vi "qc5psm.vi"() -> ()   [LabVIEW 2020]
uses:
  <instrlib>/CAEN PSM/CAEN PSM.lvlib
panel:
  in  "Tab Control":enum32{"Page 1"}(tab)
  in  "VISA resource name":refnum<visa-resource-name>
  in  "Serial Configuration":T1={"Baud Rate"=9600, "Parity"=enum."None", "Data Bits"=8, "Stop Bits"=10, "Flow Control"=0} {"Flow Control" items=["None", "XON/XOFF", "RTS/CTS", "XON/XOFF & RTS/CTS", "DTR/DSR", "XON/XOFF & DTR/DSR"]; "Stop Bits" items=["1.0"=10, "1.5"=15, "2.0"=20]; "Data Bits" items=["7"=7, "8"=8]; "Baud Rate" items=["300"=300, "600"=600, "1200"=1200, "2400"=2400, "4800"=4800, "9600"=9600, "19200"=19200, "38400"=38400, "57600"=57600, "115200"=115200]}
  in  "Voltage ramp up (0 V/s)":u16 max=999
  in  "Voltage Max (0.0 V)":u16 max=9999
  in  "Board Address":i8 max=31
  in  "Vset":dbl
  out "OVV 2":bool
  out "OVC 2":bool
  out "V monitor 2":dbl(graph)
  out "I monitor 2":dbl(graph)
  out "R calc 2":dbl
  out "Actual current level (Imon) 2":dbl
  out "Actual voltage level (Vmon) 2":dbl
  in  "START AGAIN":bool
  out "Channel Status Array":T2(array[cluster])
  in  "Channel (0)":u8
  in  "Req (Mohm)":dbl
  in  "CLOSE":bool
  out "I set status 3":dbl
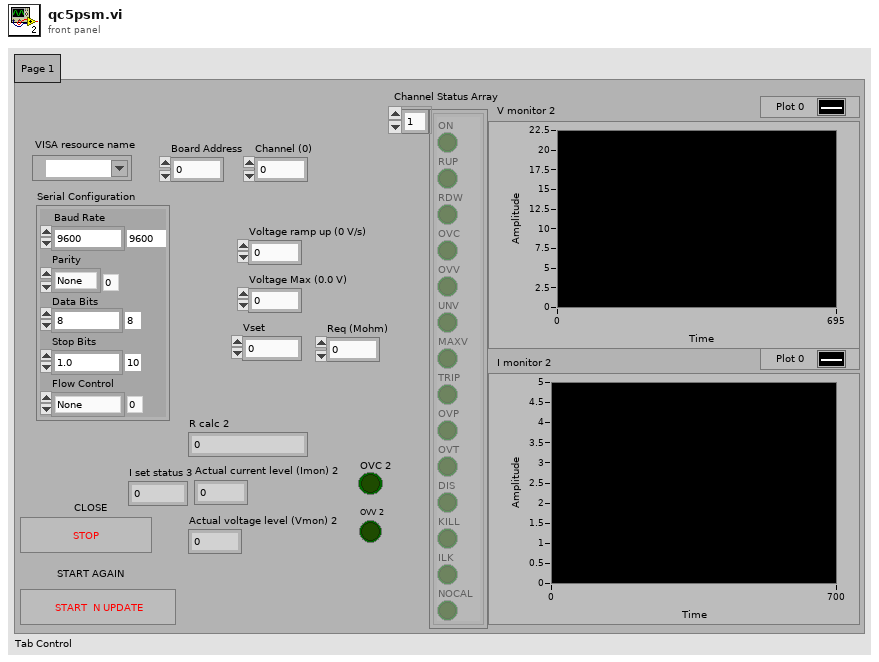
[diagram p1: front panel]
types:
  T1 = cluster{"Baud Rate":u32, "Parity":enum16{"None", "Odd", "Even", "Mark", "Space"}, "Data Bits":u16, "Stop Bits":u16, "Flow Control":u16}
  T2 = cluster{"ON":bool, "RUP":bool, "RDW":bool, "OVC":bool, "OVV":bool, "UNV":bool, "MAXV":bool, "TRIP":bool, "OVP":bool, "OVT":bool, "DIS":bool, "KILL":bool, "ILK":bool, "NOCAL":bool}[]
  T3 = typedef "CAEN PSM.lvlib/BoardHandle.ctl" = cluster{"VISA resource name":refnum<visa-resource-name>, "Board address":i8, "NChannels":u8}
  T4 = cluster{"ON":bool, "RUP":bool, "RDW":bool, "OVC":bool, "OVV":bool, "UNV":bool, "MAXV":bool, "TRIP":bool, "OVP":bool, "OVT":bool, "DIS":bool, "KILL":bool, "ILK":bool, "NOCAL":bool}
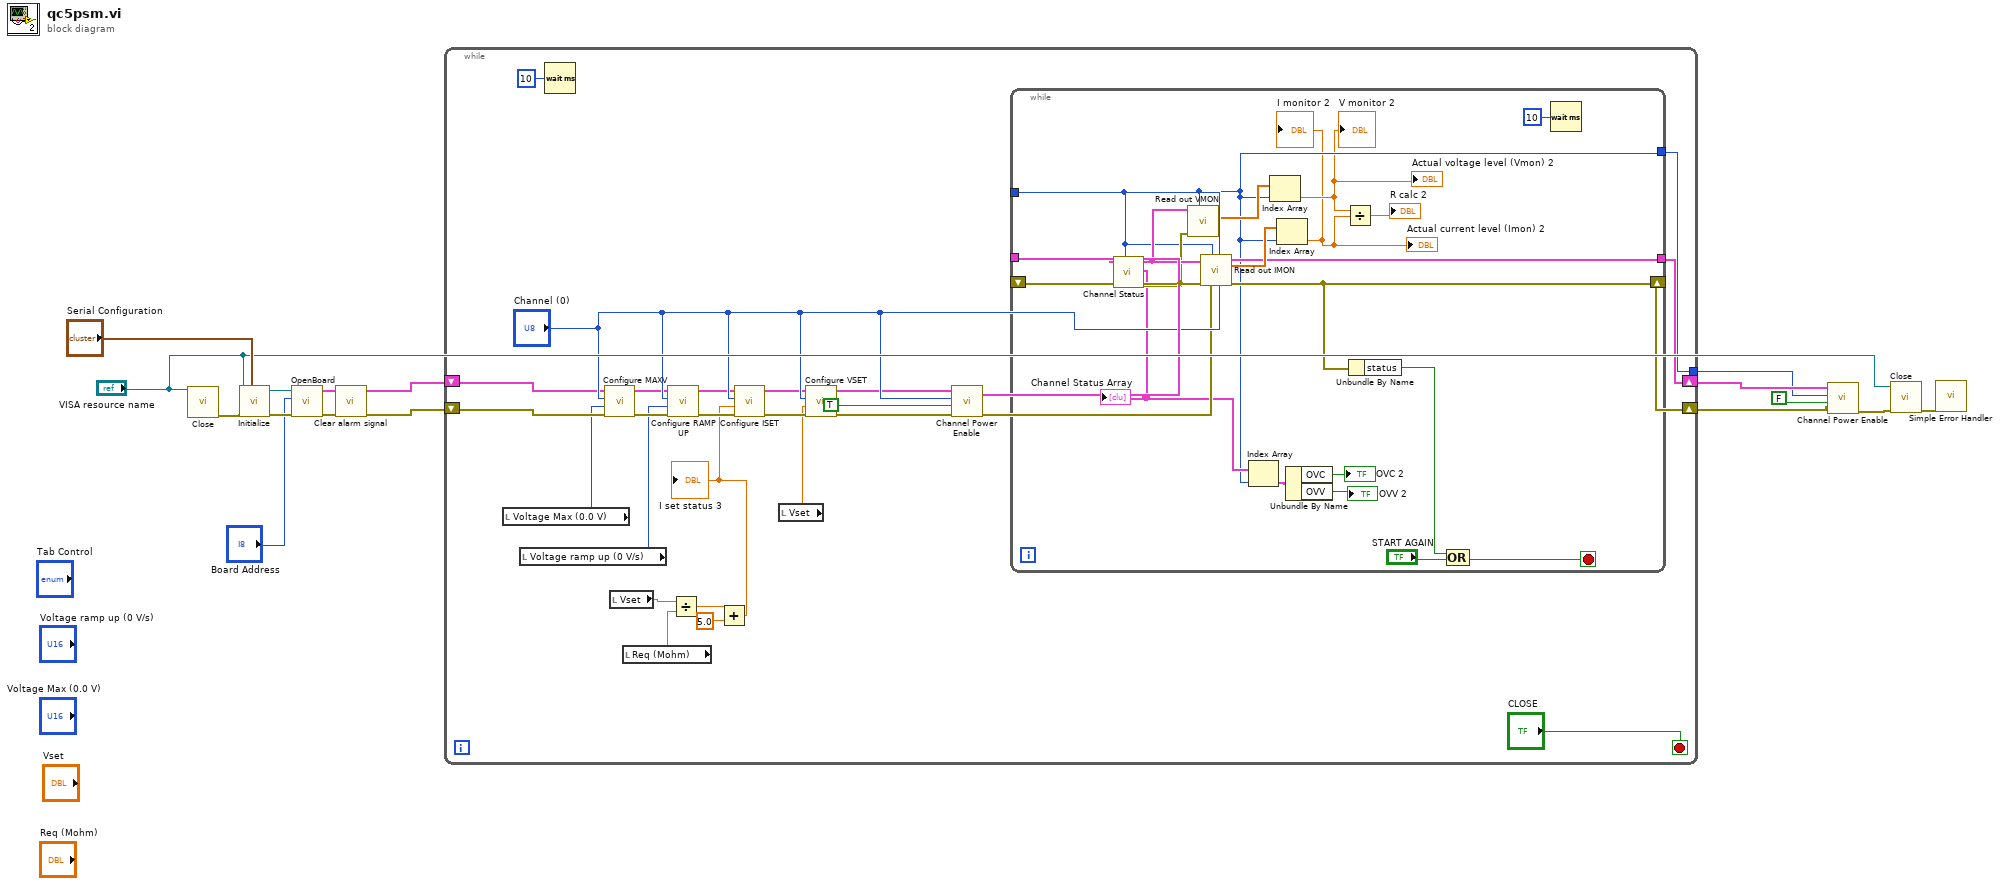
[diagram p0: block diagram]
diagram:
  n1 = call <instrlib>:"Close.vi"("VISA resource name"="VISA resource name") -> ("error out"=w8:errorcluster)  [unwired: 10 in]
  n2 = call <instrlib>:"Initialize.vi"("Serial Configuration"="Serial Configuration", "error in (no error)"=w8, "VISA resource name"="VISA resource name") -> ("error out"=w15:errorcluster, "VISA resource name out"=w14:refnum<visa-resource-name>)  [unwired: 7 in]
  n3 = call <instrlib>:"OpenBoard.vi"("error in (no error)"=w15, "Board Address"="Board Address", "VISA resource name"=w14) -> ("error out"=w12:errorcluster, "BoardHandle"=w13:T3)  [unwired: 7 in]
  n4 = call <instrlib>:"Clear alarm signal.vi"("error in (no error)"=w12, "BoardHandle"=w13) -> ("error out"=w2:errorcluster, "BoardHandle out"=w3:T3)  [unwired: 8 in]
  n5 = while {
    tunnel: [w42] -> w4
    shift-right: [w43] -> w5
    shift-left: w3 -> [w39]
    shift-right: [w24] -> w1
    shift-left: w2 -> [w38]
    stop <- "CLOSE" stop-if-true
    n6 = local read "Voltage Max (0.0 V)"() -> (w35:u16)
    n7 = local read "Voltage ramp up (0 V/s)"() -> (w34:u16)
    n8 = Wait (ms)(milliseconds to wait=u32 10) -> ()  [unwired: 1 out]
    n9 = call <instrlib>:"Configure MAXV.vi"("error in (no error)"=w38, "Voltage Max (0.0 V)"=w35, "Channel (0)"="Channel (0)", "BoardHandle"=w39) -> ("error out"=w36:errorcluster, "BoardHandle out"=w37:T3)  [unwired: 6 in]
    n10 = local read "Vset"() -> (w21:dbl)
    n11 = local read "Req (Mohm)"() -> (w20:dbl)
    n12 = call <instrlib>:"Configure RAMP UP.vi"("error in (no error)"=w36, "Voltage ramp up (0 V/s)"=w34, "Channel (0)"="Channel (0)", "BoardHandle"=w37) -> ("error out"=w29:errorcluster, "BoardHandle out"=w32:T3)  [unwired: 6 in]
    n13 = Divide(x=w21, y=w20) -> (x/y=w23:dbl)
    n14 = Add(x=w23, y=5.0) -> (x+y=w19:dbl)
    "I set status 3" <- w19
    n15 = call <instrlib>:"Configure ISET.vi"("error in (no error)"=w29, "Current Limit (0.00 uA)"=w19, "Channel (0)"="Channel (0)", "BoardHandle"=w32) -> ("error out"=w28:errorcluster, "BoardHandle out"=w30:T3)  [unwired: 6 in]
    n16 = local read "Vset"() -> (w26:dbl)
    n17 = call <instrlib>:"Configure VSET.vi"("error in (no error)"=w28, "Voltage Level (0.0 V)"=w26, "Channel (0)"="Channel (0)", "BoardHandle"=w30) -> ("error out"=w27:errorcluster, "BoardHandle out"=w31:T3)  [unwired: 6 in]
    n18 = call <instrlib>:"Channel Power Enable.vi"("error in (no error)"=w27, "Enable (OFF)"=TRUE, "Channel (0)"="Channel (0)", "BoardHandle"=w31) -> ("error out"=w25:errorcluster, "BoardHandle out"=w41:T3)  [unwired: 6 in]
    n19 = while {
      shift-right: [w53] -> w24
      shift-left: w25 -> [w44]
      tunnel: [w51] -> w43
      tunnel: [w50] -> w42
      tunnel: w41 -> [w45]
      tunnel: "Channel (0)" -> [w50]
      stop <- w56 stop-if-true
      n20 = call <instrlib>:"Channel Status.vi"("Channel"=w50, "error in (no error)"=w44, "BoardHandle"=w45) -> ("error out"=w62:errorcluster, "Channel Status Array"=w60:T2, "BoardHandle out"=w63:T3)  [unwired: 5 in, 1 out]
      "Channel Status Array" <- w60
      n21 = call <instrlib>:"Read out VMON.vi"("Channel"=w50, "error in (no error)"=w62, "BoardHandle"=w63) -> ("VMon values (V)"=w61:dbl[])  [unwired: 6 in, 2 out]
      n22 = call <instrlib>:"Read out IMON.vi"("Channel"=w50, "error in (no error)"=w62, "BoardHandle"=w63) -> ("error out"=w53:errorcluster, "IMon values (uA)"=w52:dbl[], "BoardHandle out"=w51:T3)  [unwired: 5 in, 1 out]
      n23 = Index Array(array=w60, index=w50) -> (element=w59:T4)
      n24 = Index Array(array=w61, index=w50) -> (element=w49:dbl)
      "Actual voltage level (Vmon) 2" <- w49
      "V monitor 2" <- w49
      n25 = Index Array(array=w52, index=w50) -> (element=w48:dbl)
      "Actual current level (Imon) 2" <- w48
      "I monitor 2" <- w48
      n26 = Unbundle By Name(w59) -> ("OVC"=→"OVC 2":bool, "OVV"=→"OVV 2":bool)
      n27 = Divide(x=w49, y=w48) -> (x/y=→"R calc 2":dbl)
      n28 = Unbundle By Name(w53) -> ("status"=w55:bool)
      n29 = Compound Arithmetic op=OR(w55, "START AGAIN") -> (w56:bool)
      n30 = Wait (ms)(milliseconds to wait=u32 10) -> ()  [unwired: 1 out]
    }
  }
  n31 = call <instrlib>:"Channel Power Enable.vi"("error in (no error)"=w1, "Enable (OFF)"=FALSE, "Channel (0)"=w4, "BoardHandle"=w5) -> ("error out"=w10:errorcluster)  [unwired: 6 in, 1 out]
  n32 = call <instrlib>:"Close.vi"("error in (no error)"=w10, "VISA resource name"="VISA resource name") -> ("error out"=w9:errorcluster)  [unwired: 9 in]
  n33 = call <vilib>:"Simple Error Handler.vi"("error in (no error)"=w9) -> ()  [unwired: 4 in, 5 out]
